vi "CheckSRnumber(SubVI).vi"(8 "error in (no error)":errorcluster, 11 "Data In":string[](array[string])) -> (0 "error out":errorcluster, 2 "Valid ?":bool, 3 "Data Out":string[](array[string]))   [LabVIEW 2017, in "Data Operations.lvlib"]
uses:
  Data Operations.lvlib
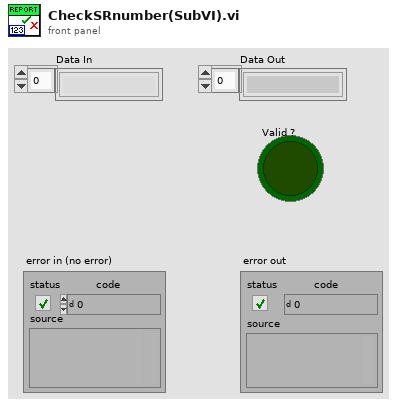
[diagram p1: front panel]
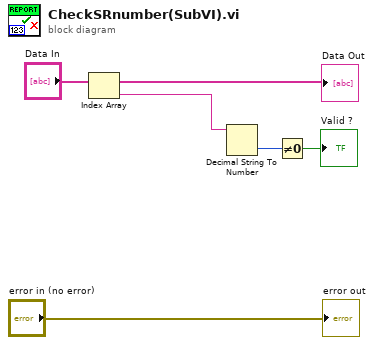
[diagram p0: block diagram]
diagram:
  n1 = Index Array(array="Data In") -> (element=w5:string)  [unwired: 1 in]
  n2 = Decimal String To Number(string=w5) -> (number=w2:i32)  [unwired: 2 in, 1 out]
  n3 = Not Equal To 0?(x=w2) -> (x != 0?=→"Valid ?":bool)
  "Data Out" <- "Data In"
  "error out" <- "error in (no error)"
